vi "CreateHardwareLogString.vi"(11 "Hardware Log Data Queue Elements":T1[](array[typedef])) -> (3 "Hardware Log String":string)   [LabVIEW 2012]
uses:
  HardwareLogData.ctl
  HardwareDisplayData.ctl
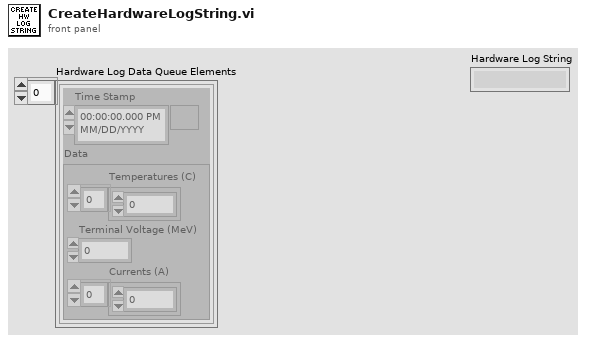
[diagram p1: front panel]
types:
  T1 = typedef "HardwareLogData.ctl" = cluster{"Time Stamp":timestamp, "Data":T2}
  T2 = typedef "HardwareDisplayData.ctl" = cluster{"Temperatures (C)":dbl[], "Terminal Voltage (MeV)":dbl, "Currents (A)":dbl[]}
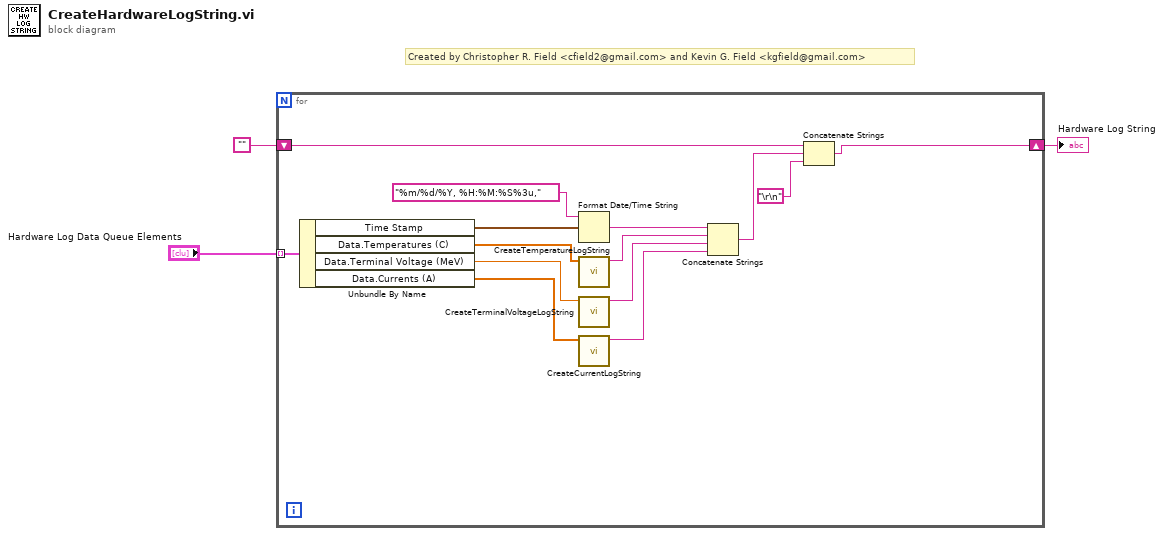
[diagram p0: block diagram]
diagram:
  # "Created by Christopher R. Field <cfield2@gmail.com> and Kevin G. Field <kgfield@gmail.com>"
  n1 = for {
    tunnel: "Hardware Log Data Queue Elements" -> [w17] mode=indexing
    shift-right: [w9] -> w1
    shift-left: "" -> [w12]
    n2 = Unbundle By Name(w17) -> ("Time Stamp"=w16:timestamp, "Data.Temperatures (C)"=w13:dbl[], "Data.Terminal Voltage (MeV)"=w7:dbl, "Data.Currents (A)"=w5:dbl[])
    n3 = Format Date/Time String(time format string (%c)="%m/%d/%Y, %H:%M:%S%3u,", seconds (now)=w16) -> (date/time string=w14:string)  [unwired: 1 in]
    n4 = call "CreateTemperatureLogString.vi"("Temperatures (C)"=w13) -> ("Temperature Log String"=w8:string)  [unwired: 10 in]
    n5 = call "CreateTerminalVoltageLogString.vi"("Terminal Voltage (MeV)"=w7) -> ("Terminal Voltage Log String"=w6:string)  [unwired: 10 in]
    n6 = call "CreateCurrentLogString.vi"("Currents (A)"=w5) -> ("Currents Log String"=w4:string)  [unwired: 10 in]
    n7 = Concatenate Strings(w14, w8, w6, w4) -> (w11:string)
    n8 = Concatenate Strings(w12, w11, "\r\n") -> (w9:string)
  }
  "Hardware Log String" <- w1
